vi "IPC-Modbus-Transfer-DecodeRequest-ReadCoils.vi"(4 "无符号字节数组":u8[](array[numeric])) -> (1 "Read coils request":T1)   [LabVIEW 2014]
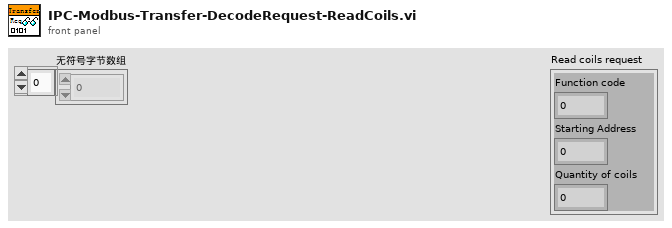
[diagram p1: front panel]
types:
  T1 = cluster{"Function code":u8, "Starting Address":u16, "Quantity of coils":u16}
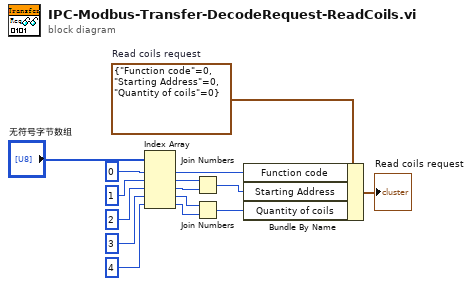
[diagram p0: block diagram]
diagram:
  w14 = T1 {"Function code"=0, "Starting Address"=0, "Quantity of coils"=0}  # Read coils request
  n1 = Index Array(array="无符号字节数组", index #1=0 ("索引"), index #2=1 ("索引"), index #3=2 ("索引"), index #4=3 ("索引"), index #5=4 ("索引")) -> (element #1=w8:u8, element #2=w7:u8, element #3=w6:u8, element #4=w4:u8, element #5=w3:u8)
  n2 = Join Numbers(hi=w7, lo=w6) -> ((hi.lo)=w5:u16)
  n3 = Join Numbers(hi=w4, lo=w3) -> ((hi.lo)=w2:u16)
  n4 = Bundle By Name(cluster=w14, "Function code"=w8, "Starting Address"=w5, "Quantity of coils"=w2) -> (→"Read coils request":T1)
